vi "DecodeSensorBytes2Floats.vi"(8 "error in":errorcluster, 11 "VISA resource name":refnum<visa-resource-name>) -> (0 "error out":errorcluster, 3 "VISA resource name out":refnum<visa-resource-name>, 5 "Array":sgl[][](array[numeric]), 7 "Bytes":u32)   [LabVIEW 2010]
panel:
  out "Received In":u8[](array[numeric]) format="%.0x"
  out "Received Left Over":u8[](array[numeric]) format="%.0x"
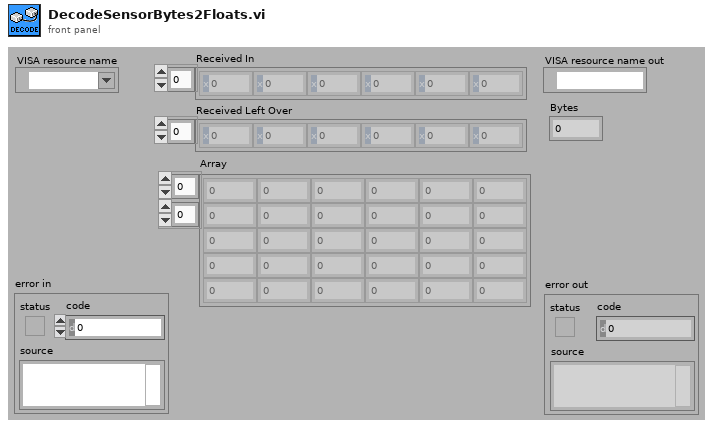
[diagram p1: front panel]
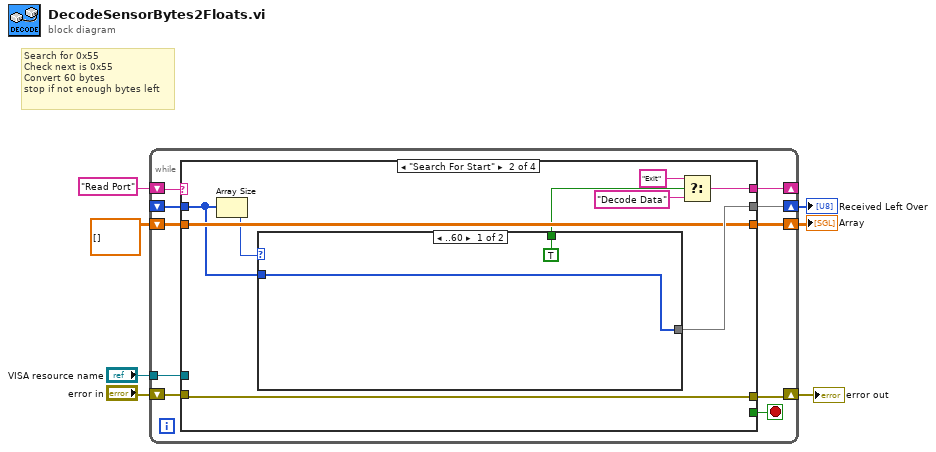
[diagram p0: block diagram]
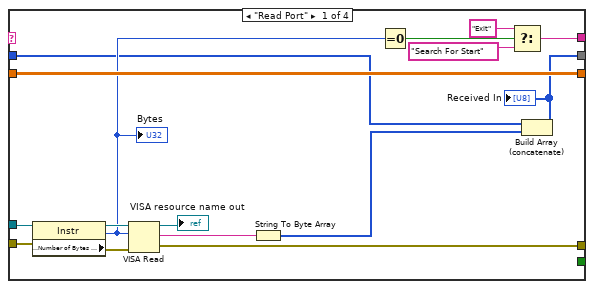
[diagram p2: hidden frame]
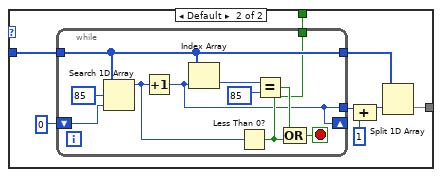
[diagram p3: hidden frame]
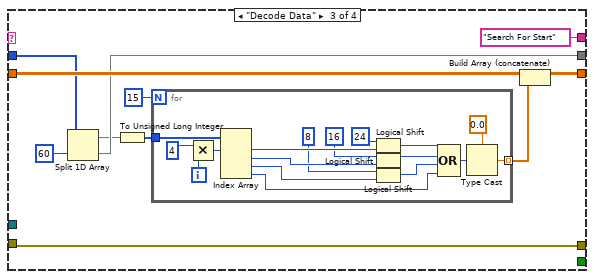
[diagram p4: hidden frame]
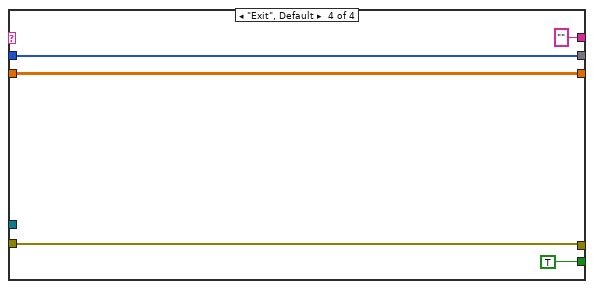
[diagram p5: hidden frame]
diagram:
  # "Search for 0x55\nCheck next is 0x55\nConvert 60 bytes\nstop if not enough bytes left"
  n1 = while {
    shift-right: [w12] -> _
    shift-left: "Read Port" -> [w17]
    tunnel: "VISA resource name" -> [w15]
    shift-right: [w13] -> w4
    shift-left: "error in" -> [w14]
    shift-right: [w11] -> w1
    shift-left: _ -> [w10]
    shift-right: [w8] -> w2
    shift-left: sgl[][] [] ("unsigned byte array") -> [w9]
    stop <- w16 stop-if-true
    n2 = case shown="\"Search For Start\"" w17 {
      tunnel: [_ _ _ TRUE] -> w16
      tunnel: w15 -> [w30 _ _ _]
      tunnel: [w28 w42 w69 w94] -> w13
      tunnel: w14 -> [w29 w42 w69 w94]
      tunnel: [w21 w35 "Search For Start" ""] -> w12
      tunnel: [w18 w41 w67 w92] -> w11
      tunnel: w10 -> [w19 w39 w70 w92]
      tunnel: w9 -> [w27 w40 w73 w91]
      tunnel: [w27 w40 w72 w91] -> w8
      frame "Read Port" {
        n3 = property class="Instr"(reference=w30, error in=w29) -> (reference out=w32:refnum<visa-resource-name>, error out=w33:errorcluster, "Serial Settings:Number of Bytes at Serial Port"=w22:u32)
        "Bytes" <- w22
        n4 = VISA Read(VISA resource name=w32, byte count=w22, error in (no error)=w33) -> (VISA resource name out=→"VISA resource name out":refnum<visa-resource-name>, read buffer=w31:string, error out=w28:errorcluster)  [unwired: 1 out]
        n5 = String To Byte Array(string=w31) -> (unsigned byte array=w20:u8[])
        n6 = Equal To 0?(x=w22) -> (x = 0?=w23:bool)
        n7 = Select(t="Exit", s=w23, f="Search For Start") -> (s? t:f=w21:string)
        n8 = Build Array (concatenate)(w19, w20) -> (w18:u8[])
        "Received In" <- w18
      }
      frame "Search For Start" {
        n9 = Array Size(array=w39) -> (size(s)=w38:i32)
        n10 = case shown="..60" w38 {
          tunnel: [w44 w51] -> w41
          tunnel: w39 -> [w44 w50]
          tunnel: [TRUE w46] -> w37
          frame ..60 {
          }
          frame Default {
            n11 = while {
              tunnel: [w53] -> w49
              tunnel: [w60] -> w52
              tunnel: w50 -> [w60]
              tunnel: [w55] -> w46
              shift-right: [w53] -> _
              shift-left: 0 -> [w54]
              stop <- w57 stop-if-true
              n12 = Search 1D Array(1D array=w60, element=u8 85, start index (0)=w54) -> (index of element=w56:i32)
              n13 = Increment(x=w56) -> (x+1=w53:i32)
              n14 = Index Array(array=w60, index=w53) -> (element=w61:u8)
              n15 = Less Than 0?(x=w56) -> (x < 0?=w55:bool)
              n16 = Equal?(x=w61, y=u8 85 ("element")) -> (x = y?=w58:bool)
              n17 = Compound Arithmetic op=OR(w58, w55) -> (w57:bool)
            }
            n18 = Compound Arithmetic op=ADD(w49, 1 ("value")) -> (w48:i32)
            n19 = Split 1D Array(array=w52, index=w48) -> (second subarray=w51:u8[])  [unwired: 1 out]
          }
        }
        n20 = Select(t="Exit", s=w37, f="Decode Data") -> (s? t:f=w35:string)
      }
      frame "Decode Data" {
        n21 = Split 1D Array(array=w70, index=60) -> (first subarray=w63:u8[], second subarray=w67:u8[])
        n22 = To Unsigned Long Integer(number=w63) -> (unsigned 32bit integer=w66:u32[])
        n23 = for {
          N: 15 -> [_]
          tunnel: w66 -> [w89]
          tunnel: [w74] -> w65 mode=indexing
          i -> [w78]
          n24 = Multiply(x=4, y=w78) -> (x*y=w79:i32)
          n25 = Index Array(array=w89, index #1=w79) -> (element #1=w90:u32, element #2=w87:u32, element #3=w86:u32, element #4=w80:u32)  [unwired: 3 in]
          n26 = Logical Shift(y=i16 24, x=w90) -> (x << y=w83:u32)
          n27 = Logical Shift(y=i16 16, x=w87) -> (x << y=w82:u32)
          n28 = Logical Shift(y=i16 8, x=w86) -> (x << y=w81:u32)
          n29 = Compound Arithmetic op=OR(w83, w82, w81, w80) -> (w75:u32)
          n30 = Type Cast(type=sgl 0.0, x=w75) -> (*(type *) &x=w74:sgl)
        }
        n31 = Build Array (concatenate)(w73, w65) -> (w72:sgl[][])
      }
      frame "Exit", Default {
      }
    }
  }
  "error out" <- w4
  "Array" <- w2
  "Received Left Over" <- w1
